vi "Get Cluster Refnum.vi"(0 "Controls[]":refnum<vi>[](array[refnum]), 11 "error in (no error)":errorcluster) -> (4 "Config":refnum<vi>, 6 "Results":refnum<vi>, 15 "error out":errorcluster)   [LabVIEW 2021, in "Measurement Client.lvlib"]
uses:
  Measurement Client.lvlib
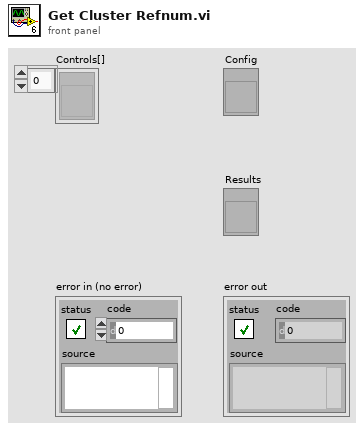
[diagram p1: front panel]
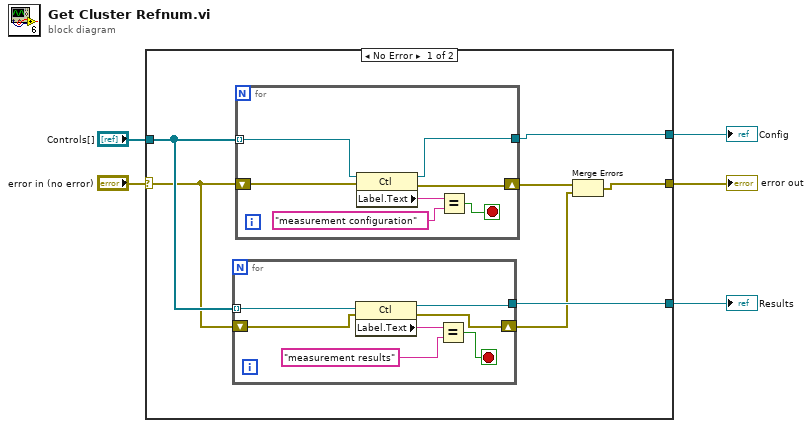
[diagram p0: block diagram]
diagram:
  n1 = case shown="No Error" "error in (no error)" {
    selector: "error in (no error)" -> [w11 w27]
    tunnel: [w7 w27] -> w5
    tunnel: "Controls[]" -> [w12 _]
    tunnel: [w10 _] -> w2
    tunnel: [w9 _] -> w1
    frame No Error {
      n2 = for {
        tunnel: w12 -> [w17] mode=indexing
        tunnel: [w14] -> w9
        shift-right: [w13] -> w6
        shift-left: w11 -> [w18]
        stop <- w15 stop-if-true
        n3 = property class="Ctl"(reference=w17, error in=w18) -> (reference out=w14:refnum<vi>, error out=w13:errorcluster, "Label.Text"=w19:string)
        n4 = Equal?(x=w19, y="measurement results") -> (x = y?=w15:bool)
      }
      n5 = for {
        tunnel: w12 -> [w26] mode=indexing
        tunnel: [w22] -> w10
        shift-right: [w21] -> w8
        shift-left: w11 -> [w25]
        stop <- w20 stop-if-true
        n6 = property class="Ctl"(reference=w26, error in=w25) -> (reference out=w22:refnum<vi>, error out=w21:errorcluster, "Label.Text"=w24:string)
        n7 = Equal?(x=w24, y="measurement configuration") -> (x = y?=w20:bool)
      }
      n8 = Merge Errors(w8, w6) -> (w7:errorcluster)
    }
    frame Error {
    }
  }
  "error out" <- w5
  "Config" <- w2
  "Results" <- w1
